vi "New Assert Message.vi"(8 "error in (no error)":errorcluster, 10 "Assert Message":T1, 11 "Standard Display Configuration in":refnum<class "Standard Display Configuration.lvclass">) -> (0 "error out":errorcluster, 3 "Standard Display Configuration out":refnum<class "Standard Display Configuration.lvclass">)   [LabVIEW 2016, in "Assert API Components.lvlib" / "Assert Display.lvlib" / "Main Display.lvlib" / "Standard Display Configuration.lvclass"]
uses:
  Standard Display Configuration.lvclass
  Assert API Components/Message Data.ctl
  Assert API Components/VI References.ctl
  Standard Display Configuration.lvclass/Standard Display Configuration.ctl
  Assert API Components/Assert API Components.lvlib
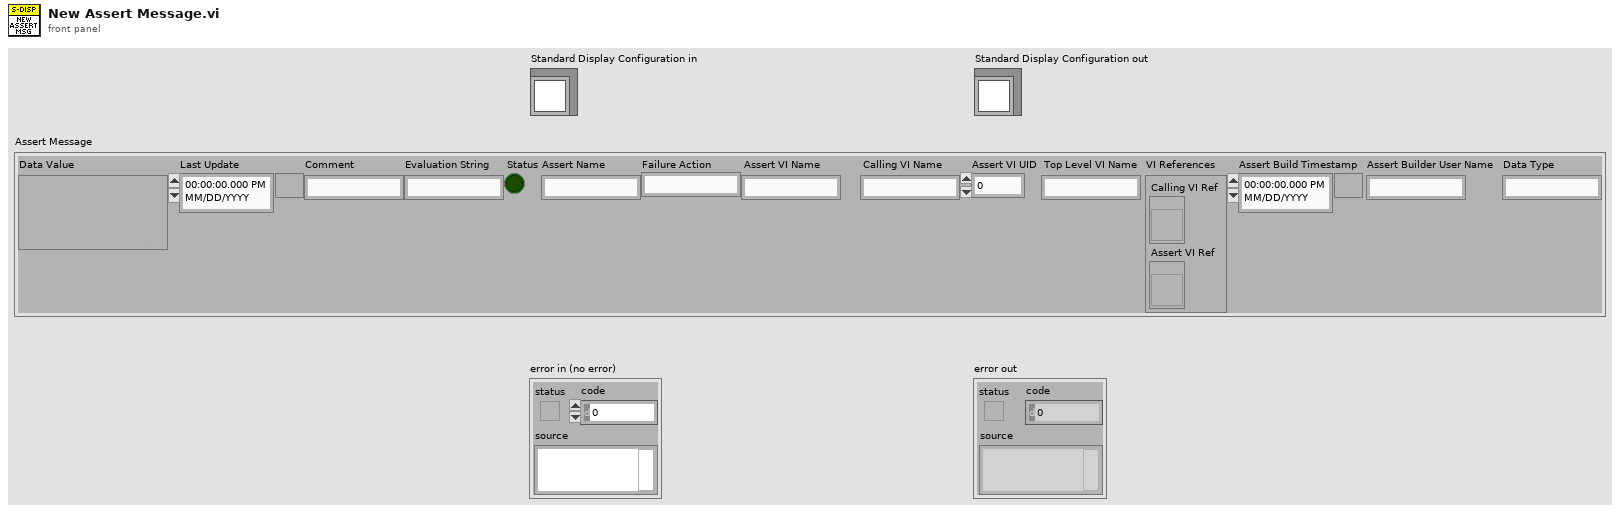
[diagram p1: front panel]
types:
  T1 = typedef "Assert API Components.lvlib/Message Data.ctl" = cluster{"Data Value":variant, "Last Update":timestamp, "Comment":string, "Evaluation String":string, "Status":bool, "Assert Name":string, "Failure Action":string, "Assert VI Name":string, "Calling VI Name":string, "Assert VI UID":i32, "Top Level VI Name":string, "VI References":T2, "Assert Build Timestamp":timestamp, "Assert Builder User Name":string, "Data Type":string}
  T2 = typedef "Assert API Components.lvlib/VI References.ctl" = cluster{"Calling VI Ref":refnum<vi>, "Assert VI Ref":refnum<vi>}
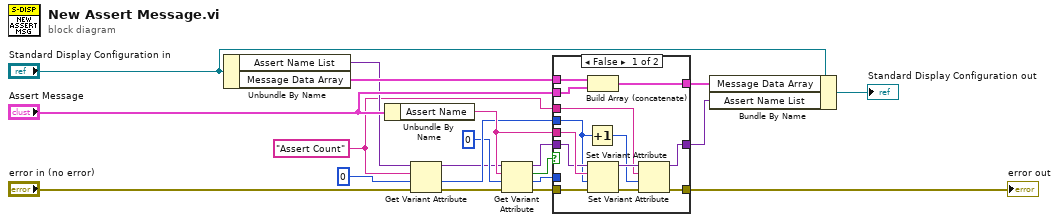
[diagram p0: block diagram]
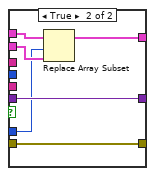
[diagram p2: hidden frame]
diagram:
  w5 = "Assert Count" ("name")
  n1 = Unbundle By Name("Standard Display Configuration in") -> ("Assert Name List"=w14:variant, "Message Data Array"=w17:T1[])
  n2 = Unbundle By Name("Assert Message") -> ("Assert Name"=w11:string)
  n3 = Get Variant Attribute(Variant=w14, name=w5, default value (empty Variant)=0, error in="error in (no error)") -> (duplicate Variant=w2:variant, value=w7:i32, error out=w3:errorcluster)  [unwired: 1 out]
  n4 = Get Variant Attribute(Variant=w2, name=w11, default value (empty Variant)=0, error in=w3) -> (duplicate Variant=w10:variant, found=w15:bool, value=w6:i32, error out=w12:errorcluster)
  n5 = case shown="False" w15 {
    tunnel: [w33 w37] -> w18
    tunnel: w17 -> [w32 w39]
    tunnel: "Assert Message" -> [w31 w38]
    tunnel: w7 -> [w21 _]
    tunnel: w12 -> [w30 w35]
    tunnel: w11 -> [w29 _]
    tunnel: w10 -> [w28 w36]
    tunnel: [w24 w36] -> w9
    tunnel: [w26 w35] -> w8
    tunnel: w6 -> [_ w34]
    tunnel: w5 -> [w23 _]
    frame False {
      n6 = Increment(x=w21) -> (x+1=w22:i32)
      n7 = Build Array (concatenate)(w32, w31) -> (w33:T1[])
      n8 = Set Variant Attribute(Variant=w28, name=w29, value=w21, error in=w30) -> (Variant out=w25:variant, error out=w27:errorcluster)  [unwired: 1 out]
      n9 = Set Variant Attribute(Variant=w25, name=w23, value=w22, error in=w27) -> (Variant out=w24:variant, error out=w26:errorcluster)  [unwired: 1 out]
    }
    frame True {
      n10 = Replace Array Subset(array=w39, new element=w38, index=w34) -> (w37:T1[])
    }
  }
  "error out" <- w8
  n11 = Bundle By Name(cluster="Standard Display Configuration in", "Message Data Array"=w18, "Assert Name List"=w9) -> (→"Standard Display Configuration out":refnum<class "Standard Display Configuration.lvclass">)
